vi "AddFooterToPNG.vi"(8 "error in (no error)":errorcluster, 10 "Footer String":string, 11 "PNG File":path) -> (0 "error out":errorcluster)   [LabVIEW 2020, in "VIDiffScreenshots.lvlib"]
uses:
  VIDiffScreenshots.lvlib
  ImageMagic/Label Position.ctl
  ImageMagic/VIDiffImageMagic.lvlib
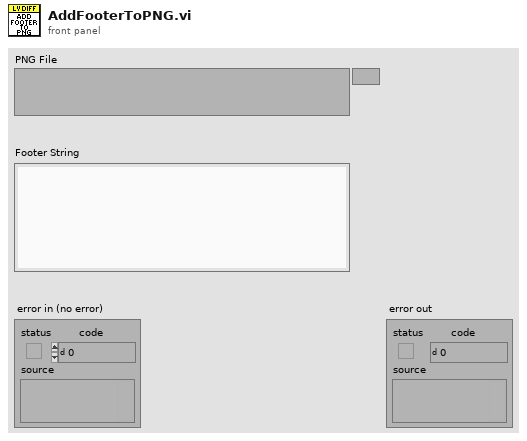
[diagram p1: front panel]
types:
  T1 = typedef "VIDiffImageMagic.lvlib/Label Position.ctl" = enum16{"Above", "Below"}
  T2 = cluster{"Font Name":string, "Size":i16, "Strikeout?":bool, "Italic?":bool, "Underline?":bool, "Bold?":bool}
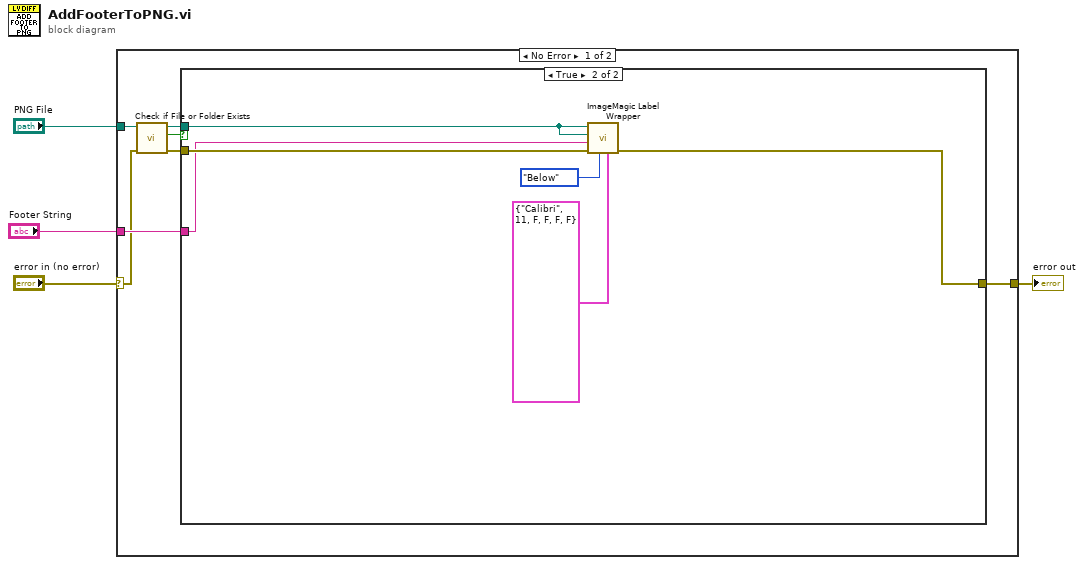
[diagram p0: block diagram]
diagram:
  n1 = case shown="No Error" "error in (no error)" {
    selector: "error in (no error)" -> [w7 w19]
    tunnel: "PNG File" -> [w9 _]
    tunnel: [w11 w19] -> w2
    tunnel: "Footer String" -> [w10 _]
    frame No Error {
      n2 = call <vilib>:"Check if File or Folder Exists.vi"("error in (no error)"=w7, "path"=w9) -> ("error out"=w8:errorcluster, "file or folder exists?"=w5:bool, "dup path"=w6:path)  [unwired: 7 in]
      n3 = case shown="True" w5 {
        tunnel: [w12 w14] -> w11
        tunnel: w10 -> [_ w15]
        tunnel: w8 -> [w12 w17]
        tunnel: w6 -> [_ w16]
        frame False {
        }
        frame True {
          n4 = call "ImageMagic Label Wrapper.vi"("Font"=T2 {"Font Name"="Calibri", "Size"=11, "Strikeout?"=FALSE, "Italic?"=FALSE, "Underline?"=FALSE, "Bold?"=FALSE}, "Label Position"=Label_Position."Below", "error in (no error)"=w17, "Text"=w15, "Output File"=w16, "Input File"=w16) -> ("error out"=w14:errorcluster)  [unwired: 5 in]
        }
      }
    }
    frame Error {
    }
  }
  "error out" <- w2
